vi "pr1b.vi"() -> ()   [LabVIEW 2013]
uses:
  <vilib>/Utility/error.llb/DialogType.ctl
  <vilib>/DAQmx/read.llb/DAQmx Read (Analog DBL 1Chan 1Samp).vi
  <vilib>/DAQmx/create/channels.llb/DAQmx Create Channel (AI-Voltage-Basic).vi
  <vilib>/DAQmx/configure/timing.llb/DAQmx Timing (Sample Clock).vi
  <vilib>/DAQmx/miscellaneous.llb/DAQmx Fill In Error Info.vi
panel:
  in  "physical channels":tag
  out "Waveform Chart":dbl(graph)
  in  "input terminal configuration":i32(ring)=-1 items=["default"=-1, "RSE"=10083, "NRSE"=10078, "Differential"=10106, "Pseudodifferential"=12529]
  in  "muestras por canal de adquisicion":i32=1000
  in  "rate m/s adquisicion":dbl=1000.0 format="%0.2f"
  in  "Valor maximo adquisicion":dbl=10.0 format="%0.2f"
  in  "Valor minimo adquisicion":dbl=-10.0 format="%0.2f"
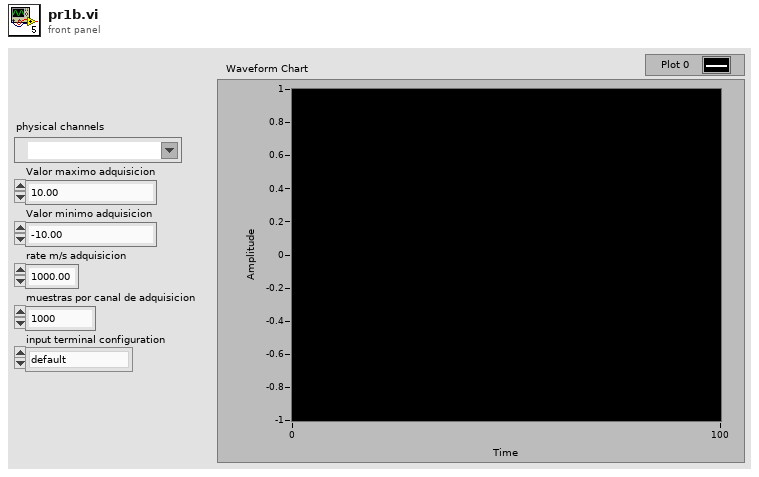
[diagram p1: front panel]
types:
  T1 = typedef "DialogType.ctl" = u16
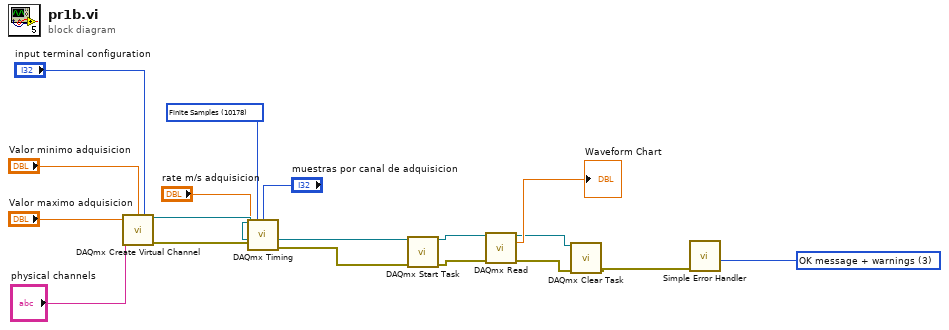
[diagram p0: block diagram]
diagram:
  w13 = T1 3 items=["no dialog", "OK message", "continue or stop message", "OK message + warnings", "continue/stop + warnings"] ("type of dialog (OK msg:1)")
  w17 = 10178 items=["Finite Samples"=10178, "Continuous Samples"=10123, "Hardware Timed Single Point"=12522] ("sample mode")
  n1 = call-poly <vilib>:"DAQmx Create Virtual Channel.vi"("maximum value"="Valor maximo adquisicion", "minimum value"="Valor minimo adquisicion", "input terminal configuration"="input terminal configuration", "physical channels"="physical channels") -> ("task out"=w18:refnum<k21>, "error out"=w16:errorcluster)  [unwired: 10 in]
  n2 = call-poly <vilib>:"DAQmx Timing.vi"("task/channels in"=w18, "sample mode"=w17, "samples per channel"="muestras por canal de adquisicion", "rate"="rate m/s adquisicion", "error in"=w16) -> ("task out"=w8:refnum<k21>, "error out"=w7:errorcluster)  [unwired: 9 in]
  n3 = call <vilib>:"DAQmx Start Task.vi"("task/channels in"=w8, "error in"=w7) -> ("task out"=w11:refnum<k21>, "error out"=w10:errorcluster)  [unwired: 12 in]
  n4 = call-poly <vilib>:"DAQmx Read.vi"("task/channels in"=w11, "error in"=w10) -> ("task out"=w2:refnum<k21>, "data"=→"Waveform Chart":dbl, "error out"=w9:errorcluster)  [unwired: 11 in]
  n5 = call <vilib>:"DAQmx Clear Task.vi"("task in"=w2, "error in"=w9) -> ("error out"=w12:errorcluster)  [unwired: 13 in]
  n6 = call <vilib>:"Simple Error Handler.vi"("type of dialog (OK msg:1)"=w13, "error in (no error)"=w12) -> ()  [unwired: 3 in, 5 out]
